vi "read_TCUStatus2.vi"(1 "Array":u8[](array[numeric])=[0, 0, 0, 0, 0, 0, 0, 0, 0, 0, 0, 0, 0, 0, 0, 0, 0, 0, 0, 0, 0, 0, 0, 0, 0, 0, 0, 0, 0, 0, 0, 0, 0, 0, 0, 0, 0, 0, 0, 0, 0, 0, 0, 0, 0, 0, 0, 0, 0, 0, 0, 0, 0, 0, 0, 0, 0, 0, 0, 0, 0, 0, 0, 0, 0, 0, 0, 0, 0, 0, 0, 0, 0, 0, 0, 0, 0, 0, 0, 0, 0, 0, 0, 0, 0, 0, 0, 0, 0, 0, 0, 0, 0, 0, 0, 0, 0, 0, 0, 0, 0, 0, 0, 0, 0, 0, 0, 0, 0, 0, 0, 0, 0, 0, 0, 0, 0, 0, 0, 0, 0, 0, 0, 0, 0, 0, 0, 0, 0, 0, 0, 0, 0, 0, 0, 0, 0, 0, 0, 0, 0, 0, 0, 0, 0, 0, 0, 0, 0, 0, 0, 0, 0, 0, 0, 0, 0, 0, 0, 0, 0, 0, 0, 0, 0, 0, 0, 0, 0, 0, 0, 0, 0, 0, 0, 0, 0, 0, 0, 0, 0]) -> (0 "output cluster":T1)   [LabVIEW 2017]
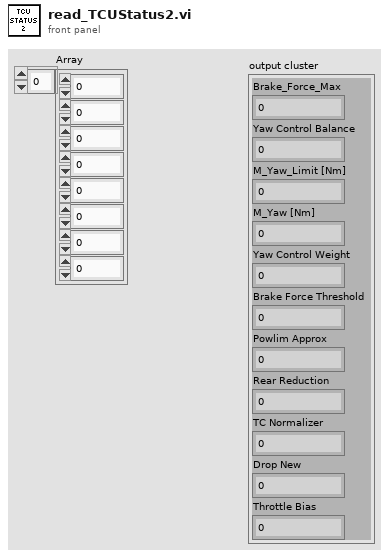
[diagram p1: front panel]
types:
  T1 = cluster{"Brake_Force_Max":u16, "Yaw Control Balance":dbl, "M_Yaw_Limit [Nm]":u16, "M_Yaw [Nm]":i16, "Yaw Control Weight":u16, "Brake Force Threshold":u16, "Powlim Approx":u16, "Rear Reduction":dbl, "TC Normalizer":u16, "Drop New":dbl, "Throttle Bias":dbl}
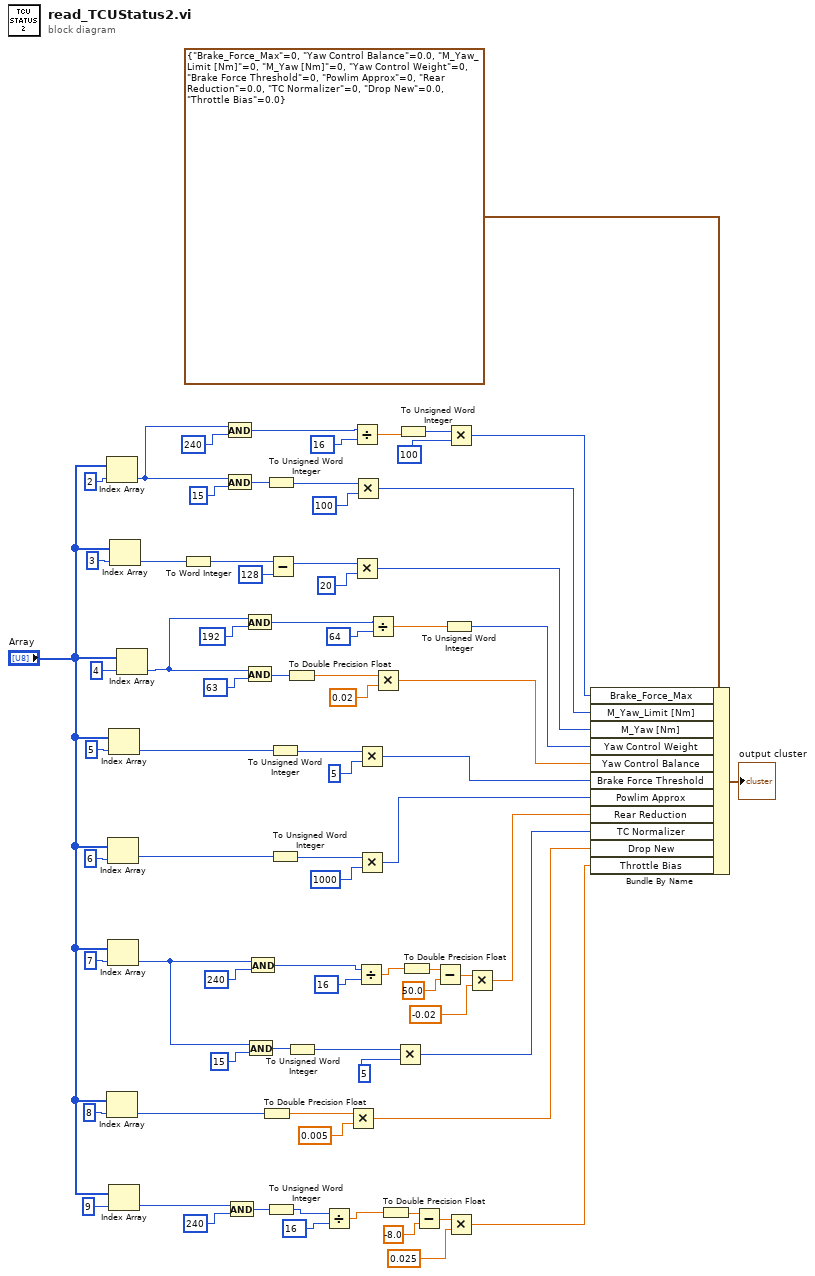
[diagram p0: block diagram]
diagram:
  n1 = Index Array(array="Array", index=2) -> (element=w64:u8)
  n2 = Index Array(array="Array", index=8) -> (element=w25:u8)
  n3 = Index Array(array="Array", index=6) -> (element=w41:u8)
  n4 = Index Array(array="Array", index=7) -> (element=w37:u8)
  n5 = Index Array(array="Array", index=5) -> (element=w44:u8)
  n6 = Index Array(array="Array", index=9) -> (element=w17:u8)
  n7 = Index Array(array="Array", index=3) -> (element=w58:u8)
  n8 = Index Array(array="Array", index=4) -> (element=w51:u8)
  n9 = To Word Integer(number=w58) -> (16bit integer=w55:i16)
  n10 = And(x=w64, y=u8 240) -> (x .and. y?=w11:u8)
  n11 = And(x=w64, y=u8 15) -> (x .and. y?=w65:u8)
  n12 = And(x=w17, y=u8 240) -> (x .and. y?=w18:u8)
  n13 = And(x=w51, y=u8 192) -> (x .and. y?=w7:u8)
  n14 = And(x=w51, y=u8 63) -> (x .and. y?=w50:u8)
  n15 = And(x=w37, y=u8 15) -> (x .and. y?=w30:u8)
  n16 = And(x=w37, y=u8 240) -> (x .and. y?=w4:u8)
  n17 = To Double Precision Float(number=w25) -> (double precision float=w27:dbl)
  n18 = To Unsigned Word Integer(number=w65) -> (unsigned 16bit integer=w67:u16)
  n19 = To Unsigned Word Integer(number=w18) -> (unsigned 16bit integer=w2:u16)
  n20 = Subtract(x=w55, y=i16 128) -> (x-y=w56:i16)
  n21 = To Unsigned Word Integer(number=w44) -> (unsigned 16bit integer=w46:u16)
  n22 = To Unsigned Word Integer(number=w41) -> (unsigned 16bit integer=w42:u16)
  n23 = To Double Precision Float(number=w50) -> (double precision float=w49:dbl)
  n24 = To Unsigned Word Integer(number=w30) -> (unsigned 16bit integer=w29:u16)
  n25 = Divide(x=w2, y=u8 16) -> (x/y=w1:dbl)
  n26 = Multiply(x=w27, y=0.005) -> (x*y=w24:dbl)
  n27 = Divide(x=w11, y=u8 16) -> (x/y=w12:dbl)
  n28 = Multiply(x=w56, y=i16 20) -> (x*y=w59:i16)
  n29 = Multiply(x=w67, y=u16 100) -> (x*y=w63:u16)
  n30 = Divide(x=w4, y=u8 16) -> (x/y=w5:dbl)
  n31 = Multiply(x=w46, y=u16 5) -> (x*y=w45:u16)
  n32 = Multiply(x=w42, y=u16 1000) -> (x*y=w40:u16)
  n33 = Divide(x=w7, y=u8 64) -> (x/y=w8:dbl)
  n34 = Multiply(x=w49, y=0.02) -> (x*y=w48:dbl)
  n35 = To Double Precision Float(number=w1) -> (double precision float=w20:dbl)
  n36 = Multiply(x=w29, y=u16 5) -> (x*y=w28:u16)
  n37 = To Unsigned Word Integer(number=w12) -> (unsigned 16bit integer=w13:u16)
  n38 = To Double Precision Float(number=w5) -> (double precision float=w36:dbl)
  n39 = Subtract(x=w20, y=-8.0) -> (x-y=w22:dbl)
  n40 = Subtract(x=w36, y=50.0) -> (x-y=w34:dbl)
  n41 = To Unsigned Word Integer(number=w8) -> (unsigned 16bit integer=w14:u16)
  n42 = Multiply(x=w13, y=u16 100) -> (x*y=w68:u16)
  n43 = Multiply(x=w22, y=0.025) -> (x*y=w16:dbl)
  n44 = Multiply(x=w34, y=-0.02) -> (x*y=w32:dbl)
  n45 = Bundle By Name(cluster=T1 {"Brake_Force_Max"=0, "Yaw Control Balance"=0.0, "M_Yaw_Limit [Nm]"=0, "M_Yaw [Nm]"=0, "Yaw Control Weight"=0, "Brake Force Threshold"=0, "Powlim Approx"=0, "Rear Reduction"=0.0, "TC Normalizer"=0, "Drop New"=0.0, "Throttle Bias"=0.0}, "Brake_Force_Max"=w68, "M_Yaw_Limit [Nm]"=w63, "M_Yaw [Nm]"=w59, "Yaw Control Weight"=w14, "Yaw Control Balance"=w48, "Brake Force Threshold"=w45, "Powlim Approx"=w40, "Rear Reduction"=w32, "TC Normalizer"=w28, "Drop New"=w24, "Throttle Bias"=w16) -> (→"output cluster":T1)
